vi "Valid Local Directory Only.vi"(8 "error in":errorcluster, 10 "Directory ref":string="Archive Directory", 11 "Path input":path) -> (0 "error out":errorcluster, 3 "Path output":path)   [LabVIEW 2012]
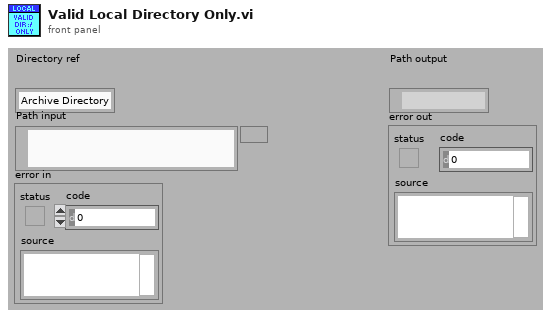
[diagram p1: front panel]
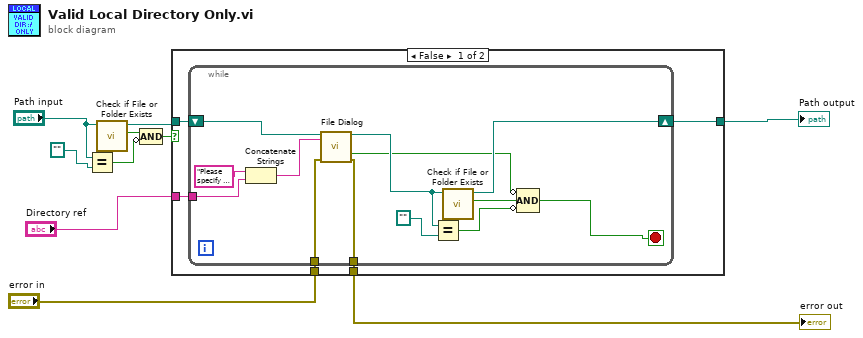
[diagram p0: block diagram]
diagram:
  n1 = Equal?(x="Path input", y=path "") -> (x = y?=w7:bool)
  n2 = call <vilib>:"Check if File or Folder Exists.vi"("path"="Path input") -> ("file or folder exists?"=w6:bool, "dup path"=w9:path)  [unwired: 8 in, 1 out]
  n3 = Compound Arithmetic op=AND(w6, invert w7) -> (w8:bool)
  n4 = case shown="False" w8 {
    tunnel: w9 -> [w15 w30]
    tunnel: [w13 w30] -> w3
    tunnel: "Directory ref" -> [w14 _]
    tunnel: "error in" -> [w12 w29]
    tunnel: [w11 w29] -> w1
    frame False {
      n5 = while {
        tunnel: w14 -> [w25]
        shift-right: [w20] -> w13
        shift-left: w15 -> [w28]
        tunnel: w12 -> [w17]
        tunnel: [w16] -> w11
        stop <- w18 stop-if-true
        n6 = Concatenate Strings("Please specify a Valid File Path for :" ("prompt"), w25) -> (w27:string)
        n7 = call "File Dialog"("start path"=w28, "prompt"=w27, "error in"=w17) -> ("selected path"=w21:path, "cancelled"=w19:bool, "error out"=w16:errorcluster)  [unwired: 9 in, 1 out]
        n8 = Equal?(x=w21, y=path "") -> (x = y?=w24:bool)
        n9 = call <vilib>:"Check if File or Folder Exists.vi"("path"=w21) -> ("file or folder exists?"=w23:bool, "dup path"=w20:path)  [unwired: 8 in, 1 out]
        n10 = Compound Arithmetic op=AND(invert w19, w23, invert w24) -> (w18:bool)
      }
    }
    frame True {
    }
  }
  "Path output" <- w3
  "error out" <- w1
